vi "Add From Spreadsheet.vi"(8 "error in (no error)":errorcluster, 10 "file path (use dialog)":path, 11 "Device BaseNodeType in":T1) -> (0 "error out":errorcluster, 1 "Address warning":bool[](array[boolean]), 3 "Device BaseNodeType out":T1)   [LabVIEW 2010, in "RefMem PtByPt Custom Device.lvlib"]
uses:
  RefMem PtByPt Custom Device.lvlib
  <vilib>/NI Veristand/Custom Device API/Custom Device Pointer.ctl
  NationalInstruments.VeriStand.SystemStorage
  Controls/Data Channel Type.ctl
  Controls/Global.vi
  <vilib>/NI Veristand/Custom Device API/Custom Device API.lvlib
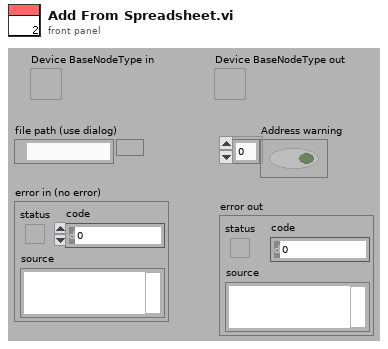
[diagram p1: front panel]
types:
  T1 = typedef "Custom Device API.lvlib/Custom Device Pointer.ctl" = refnum<k24>
  T2 = typedef "RefMem PtByPt Custom Device.lvlib/Data Channel Type.ctl" = enum16{"Read", "Write"}
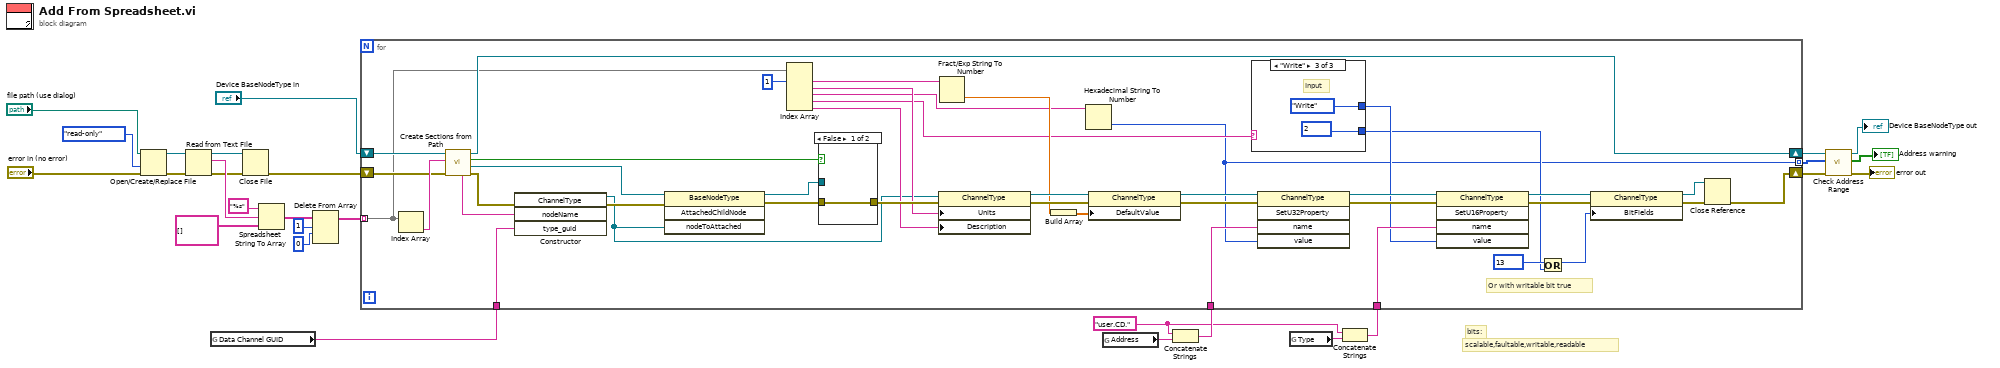
[diagram p0: block diagram]
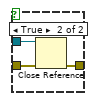
[diagram p2: hidden frame]
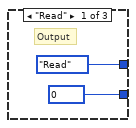
[diagram p3: hidden frame]
diagram:
  w7 = "user.CD." ("string")
  # "bits:"
  # "scalable,faultable,writable,readable"
  n1 = Open/Create/Replace File(file path (use dialog)="file path (use dialog)", error in="error in (no error)", access (0:read/write)=enum16{"read/write", "read-only", "write-only"}."read-only") -> (refnum out=w17:refnum<file>, error out=w16:errorcluster)  [unwired: 3 in, 1 out]
  n2 = Read from Text File(file (use dialog)=w17, error in=w16) -> (refnum out=w18:refnum<file>, text=w21:string, error out=w19:errorcluster)  [unwired: 2 in, 1 out]
  n3 = global read "Global.vi" "Data Channel GUID"() -> (w28:string)
  n4 = Close File(refnum=w18, error in=w19) -> (error out=w27:errorcluster)  [unwired: 1 out]
  n5 = Spreadsheet String To Array(format string="%s", spreadsheet string=w21, array type (2D Dbl)=string[][] []) -> (array=w23:string[][])  [unwired: 1 in]
  n6 = Delete From Array(array=w23, length=1, index (row)=0) -> (array with subset deleted=w26:string[][])  [unwired: 1 in, 1 out]
  n7 = global read "Global.vi" "Address"() -> (w11:string)
  n8 = Concatenate Strings(w7, w11) -> (w10:string)
  n9 = global read "Global.vi" "Type"() -> (w9:string)
  n10 = Concatenate Strings(w7, w9) -> (w8:string)
  n11 = for {
    tunnel: w26 -> [w63] mode=indexing
    shift-right: [w44] -> w5
    shift-left: w27 -> [w68]
    shift-right: [w66] -> w6
    shift-left: "Device BaseNodeType in" -> [w67]
    tunnel: w28 -> [w38]
    tunnel: w10 -> [w35]
    tunnel: w8 -> [w48]
    tunnel: [w29] -> w4 mode=indexing
    # "Or with writable bit true"
    n12 = Index Array(array=w63) -> (element=w69:string)  [unwired: 1 in]
    n13 = call "Create Sections from Path.vi"("error in"=w68, "Path"=w69, "Device BaseNodeType in"=w67) -> ("error out"=w40:errorcluster, "SectionRef"=w43:T1, "NewRef?"=w42:bool, "Device BaseNodeType out"=w66:T1, "ChannelName"=w39:string)  [unwired: 4 in]
    n14 = constructor class="ChannelType"(error in=w40, "nodeName"=w39, "type_guid"=w38) -> (reference out=w37:refnum<k24>, error out=w41:errorcluster)  [unwired: 2 in, 3 out]
    n15 = invoke class="BaseNodeType" method="AttachedChildNode"(reference=w43, error in=w41, "nodeToAttached"=w37) -> (reference out=w64:T1, error out=w65:errorcluster)  [unwired: 1 in, 2 out]
    n16 = Index Array(array=w63, index #1=1 ("index")) -> (element #1=w58:string, element #2=w59:string, element #3=w54:string, element #4=w51:string, element #5=w61:string)  [unwired: 4 in]
    n17 = case shown="False" w42 {
      tunnel: w65 -> [w70 w73]
      tunnel: w64 -> [_ w72]
      tunnel: [w70 w71] -> w62
      frame False {
      }
      frame True {
        n18 = Close Reference(reference=w72, error in (no error)=w73) -> (error out=w71:errorcluster)
      }
    }
    n19 = property class="ChannelType"(reference=w37, error in=w62, "Units"=w59, "Description"=w61) -> (reference out=w57:refnum<k24>, error out=w56:errorcluster)
    n20 = Fract/Exp String To Number(string=w58) -> (number=w55:dbl)  [unwired: 3 in, 1 out]
    n21 = Build Array(w55) -> (w36:dbl[])
    n22 = Hexadecimal String To Number(string=w54) -> (number=w29:u32)  [unwired: 2 in, 1 out]
    n23 = property class="ChannelType"(reference=w57, error in=w56, "DefaultValue"=w36) -> (reference out=w52:refnum<k24>, error out=w53:errorcluster)
    n24 = case shown="\"Write\"" w51 {
      tunnel: [Data_Channel_Type."Read" ("Type") _ Data_Channel_Type."Write" ("Type")] -> w45
      tunnel: [u32 0 ("BitFields") _ u32 2 ("BitFields")] -> w32
      frame "Read" {
        # "Output"
      }
      frame Default {
      }
      frame "Write" {
        # "Input"
      }
    }
    n25 = invoke class="ChannelType" method="SetU32Property"(reference=w52, error in=w53, "name"=w35, "value"=w29) -> (reference out=w50:refnum<k24>, error out=w49:errorcluster)  [unwired: 1 in, 3 out]
    n26 = invoke class="ChannelType" method="SetU16Property"(reference=w50, error in=w49, "name"=w48, "value"=w45) -> (reference out=w47:refnum<k24>, error out=w46:errorcluster)  [unwired: 1 in, 3 out]
    n27 = Or(x=u32 13 ("BitFields"), y=w32) -> (x .or. y?=w34:u32)
    n28 = property class="ChannelType"(reference=w47, error in=w46, "BitFields"=w34) -> (reference out=w30:refnum<k24>, error out=w31:errorcluster)
    n29 = Close Reference(reference=w30, error in (no error)=w31) -> (error out=w44:errorcluster)
  }
  n30 = call "Check Address Range.vi"("error in (no error)"=w5, "Addresses"=w4, "Node Pointer In"=w6) -> ("error out"=→"error out":errorcluster, "Inside NIVS Range"=→"Address warning":bool[], "Node Pointer dup"=→"Device BaseNodeType out":T1)  [unwired: 6 in]
